vi "Create Arbitrary Waveform.vi"(7 "Arbitrary Waveform Name (0: USER1)":u16(ring) items=["USER1", "USER2", "USER3", "USER4"], 8 "error in (no error)":errorcluster, 9 "Arbitrary Waveform Data":dbl[](array[numeric]), 11 "VISA resource name":refnum<visa-resource-name>) -> (0 "error out":errorcluster, 3 "VISA resource name out":refnum<visa-resource-name>)   [LabVIEW 2009, in "Tektronix AFG 3000 Series.lvlib"]
doc: "Creates and saves an arbitrary waveform in edit memory. \n\n<B>Note:</B>\n\nCreates an arbitrary waveform in edit memory and because of this, the waveform will remain stored on the instrument until deleted. If any sensitive information is contained in the arbitrary waveform, it is recommended that the waveform be deleted when finished."
uses:
  Tektronix AFG 3000 Series.lvlib
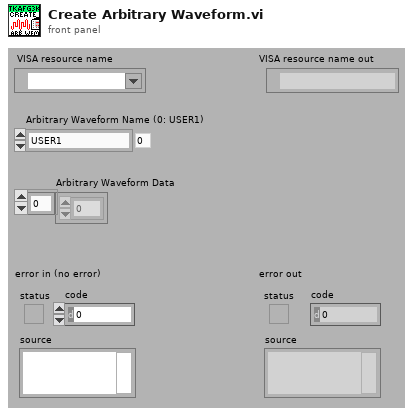
[diagram p1: front panel]
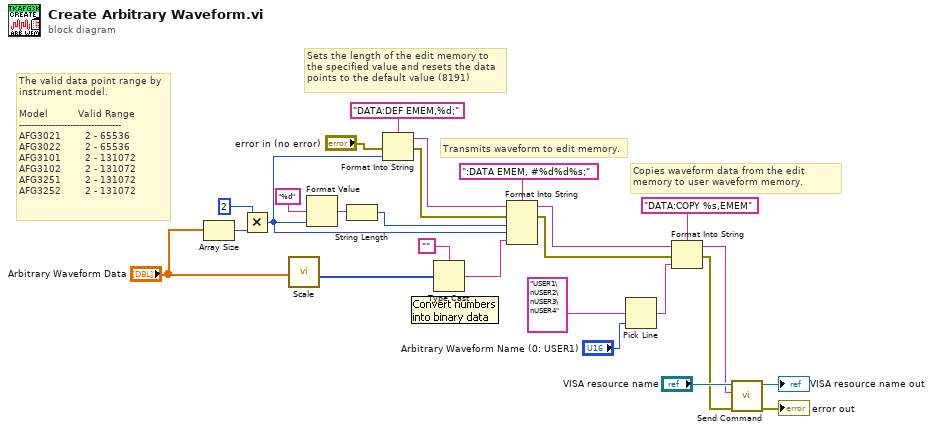
[diagram p0: block diagram]
diagram:
  # "Transmits waveform to edit memory."
  # "Sets the length of the edit memory to the specified value and resets the data points to the default value (8191)"
  # "The valid data point range by instrument model. \n\nModel          Valid Range\n----------------------------------\nAFG3021        2 - 65536\nAFG3022        2 - 65536\nAFG3101        2 - 131072\nAFG3102        2 - 131072\nAFG3251        2 - 131072\nAFG3252        2 - 131072"
  # "Copies waveform data from the edit memory to user waveform memory."
  n1 = Array Size(array="Arbitrary Waveform Data") -> (size(s)=w23:i32)
  n2 = Multiply(x=2, y=w23) -> (x*y=w11:i32)
  n3 = call "Scale.vi"("Waveform Data"="Arbitrary Waveform Data") -> ("Scaled Waveform Data"=w9:i32[])  [unwired: 2 in, 8 out]
  n4 = Format Value(format string="%d", value (0)=w11) -> (output string=w14:string)  [unwired: 1 out]
  n5 = String Length(string=w14) -> (length=w13:i32)
  n6 = Format Into String(format string="DATA:DEF EMEM,%d;", error in="error in (no error)", w11) -> (resulting string=w17:string, error out=w7:errorcluster)  [unwired: 1 in]
  n7 = Type Cast(type="", x=w9) -> (*(type *) &x=w16:string)
  n8 = Format Into String(format string=":DATA EMEM, #%d%d%s;", initial string=w17, error in=w7, w13, w11, w16) -> (resulting string=w12:string, error out=w6:errorcluster)
  n9 = Pick Line(multi-line string="USER1\nUSER2\nUSER3\nUSER4", line index="Arbitrary Waveform Name (0: USER1)") -> (output string=w19:string)  [unwired: 1 out]
  n10 = Format Into String(format string="DATA:COPY %s,EMEM", initial string=w12, error in=w6, w19) -> (resulting string=w2:string, error out=w1:errorcluster)
  n11 = call "Send Command.vi"("error in (no error)"=w1, "write buffer"=w2, "VISA resource name"="VISA resource name") -> ("error out"=→"error out":errorcluster, "VISA resource name out"=→"VISA resource name out":refnum<visa-resource-name>)  [unwired: 7 out]
